vi "PTSequencer.ProcDestructor.vi"(0 "i ref in":refnum<vi>, 5 "error in (no error)":errorcluster) -> (14 "i ref out":refnum<vi>, 19 "error out":errorcluster)   [LabVIEW 2014, in "PTSequencer.lvlib"]
uses:
  PTSequencer.lvlib
  CS_Core/BaseProcess/BaseProcess.event definition.ctl
  CS_Core/CAEObj/CAEObj.event definition.ctl
  CS_Core/BaseProcess/BaseProcess.descriptor string definition.ctl
  CSlibraries-extern/DimLVEvent/LVDimInterface/LVDimInterface.lvlib
  CS_Core/BaseProcess/BaseProcess.lvlib
  CS_Core/CAEObj/CAEObj.lvlib
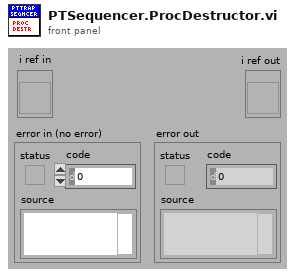
[diagram p1: front panel]
types:
  T1 = typedef "BaseProcess.lvlib/BaseProcess.event definition.ctl" = cluster{"CAEEvtDef":T2, "Data Descriptor":T3}
  T2 = typedef "CAEObj.lvlib/CAEObj.event definition.ctl" = cluster{"URL":string, "enable":bool, "ignoreResID":bool}
  T3 = typedef "BaseProcess.lvlib/BaseProcess.descriptor string definition.ctl" = string
  T4 = typedef "PTSequencer.lvlib/PTSequencer.i attribute.ctl" = cluster{"subsequence":bool, "mode":T5, "i step":i32, "nofLoops":i32, "i loop":i32, "Running":bool, "Paused":bool, "step done":bool, "loop done":bool, "seq done":bool, "DIM IDs":cluster{"step done":i32, "loop done":i32, "seq done":i32, "i step":i32, "i loop":i32}, "use stop conditions":bool, "stop conditions":T6[], "Step List":T8[], "DIM subsriptions":string[], "stop cond indexes":i32[], "step cond indexes":cluster{"step condition IDs":cluster{"step ID":i32, "condition ID":i32}[]}[], "Delay Start Time":timestamp, "status":string, "stopping":bool}
  T5 = typedef "PTSequencer.lvlib/PTSequencer.mode.ctl" = enum16{"single", "loop", "for loop"}
  T6 = typedef "PTSequencer.lvlib/PTSequencer.DIM service condition.ctl" = cluster{"DIM service":string, "descr":string, "nomValue":T7, "actValue":T7, "matched":bool, "DIM Status":cluster{"no link":bool, "quality":i32, "Time Stamp":timestamp}}
  T7 = typedef "CoreDefs.rawDataType.ctl" = i8[]
  T8 = typedef "PTSequencer.lvlib/PTSequencer.step.ctl" = cluster{"description":string, "object parameters":cluster{"object":string, "selector":string, "descriptor":string, "data":T7, "subsequence":bool, "call mode":enum16{"Simple DIM", "Synchronous"}, "data in":T7}, "result action":cluster{"check":bool, "passed":enum16{"Next", "Previous", "Repeat", "Jump"}, "failed":enum16{"Next", "Previous", "Repeat", "Jump"}, "jumpID_passed":i32, "jumpID_failed":i32}, "conditions":T6[], "fulfilled ":bool, "use delay":bool, "delay time (s)":dbl, "ID":i32}
  T9 = cluster{"step done":i32, "loop done":i32, "seq done":i32, "i step":i32, "i loop":i32}
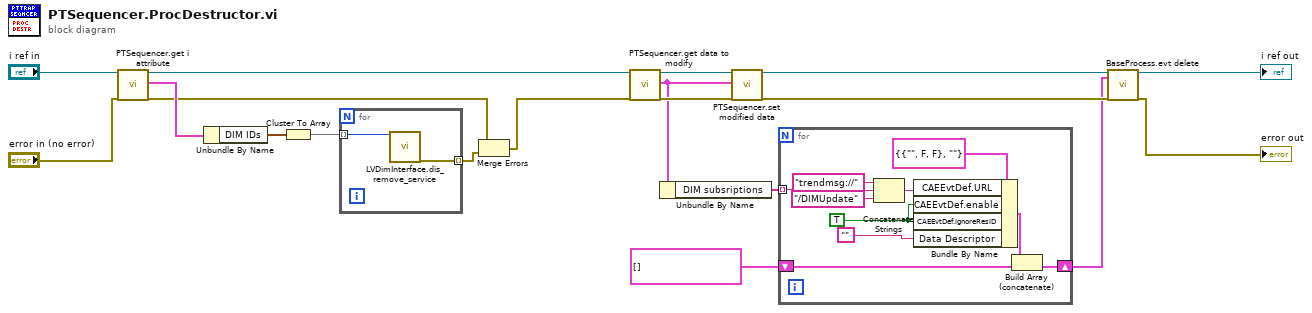
[diagram p0: block diagram]
diagram:
  n1 = call "PTSequencer.get i attribute.vi"("i ref in"="i ref in", "error in (no error)"="error in (no error)") -> ("i ref out"=w11:refnum<vi>, "i attribute"=w17:T4, "error out"=w13:errorcluster)  [unwired: 15 in]
  n2 = Unbundle By Name(w17) -> ("DIM IDs"=w16:T9)
  n3 = Cluster To Array(cluster=w16) -> (array=w15:i32[])
  n4 = for {
    tunnel: w15 -> [w21] mode=indexing
    tunnel: [w20] -> w14 mode=indexing
    n5 = call "LVDimInterface.dis_remove_service.vi"("my_serviceID"=w21) -> ("error out"=w20:errorcluster)  [unwired: 18 in]
  }
  n6 = Merge Errors(w13, w14) -> (w10:errorcluster)
  n7 = call "PTSequencer.get data to modify.vi"("i ref in"=w11, "error in (no error)"=w10) -> ("i ref out"=w7:refnum<vi>, "i attribute"=w6:T4, "error out"=w8:errorcluster)  [unwired: 14 in, 1 out]
  n8 = Unbundle By Name(w6) -> ("DIM subsriptions"=w9:string[])
  n9 = call "PTSequencer.set modified data.vi"("i ref in"=w7, "CLASS.i attribute"=w6, "error in (no error)"=w8) -> ("i ref out"=w5:refnum<vi>, "error out"=w4:errorcluster)  [unwired: 15 in]
  n10 = for {
    shift-right: [w30] -> w3
    shift-left: T1[] [] -> [w31]
    tunnel: w9 -> [w22] mode=indexing
    w25 = TRUE ("CAEEvtDef.ignoreResID")
    n11 = Concatenate Strings("trendmsg://", w22, "/DIMUpdate" ("string")) -> (w26:string)
    n12 = Bundle By Name(cluster=T1 {"CAEEvtDef"={"URL"="", "enable"=FALSE, "ignoreResID"=FALSE}, "Data Descriptor"=""} ("event definition"), "CAEEvtDef.URL"=w26, "CAEEvtDef.enable"=w25, "CAEEvtDef.ignoreResID"=w25, "Data Descriptor"="") -> (w23:T1)
    n13 = Build Array (concatenate)(w23, w31) -> (w30:T1[])
  }
  n14 = call "BaseProcess.evt delete.vi"("i ref in"=w5, "events"=w3, "error in (no error)"=w4) -> ("i ref out"=→"i ref out":refnum<vi>, "error out"=→"error out":errorcluster)  [unwired: 13 in, 2 out]
